vi "Create String for Cluster in Result.vi"(0 "vi reference":refnum<vi>, 2 "output clusters in":string[](array[string]), 5 "ctl refnum":refnum<vi>, 7 "result cluster":refnum<vi>, 11 "error in":errorcluster) -> (4 "output clusters out":string[](array[string]), 15 "error out":errorcluster)   [LabVIEW 2021, in "Converter.lvlib"]
uses:
  Converter.lvlib
  <vilib>/Utility/miscctls.llb/LVPositionTypeDef.ctl
  Converter Reusables/Converter Reusables.lvlib
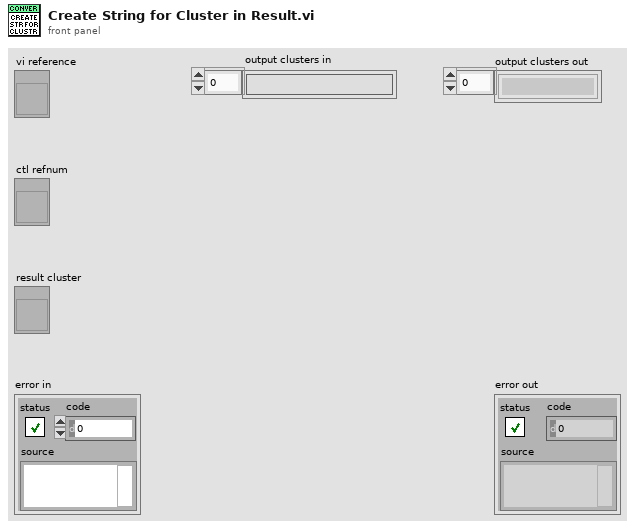
[diagram p1: front panel]
types:
  T1 = typedef "LVPositionTypeDef.ctl" = cluster{"Left":i32, "Top":i32}
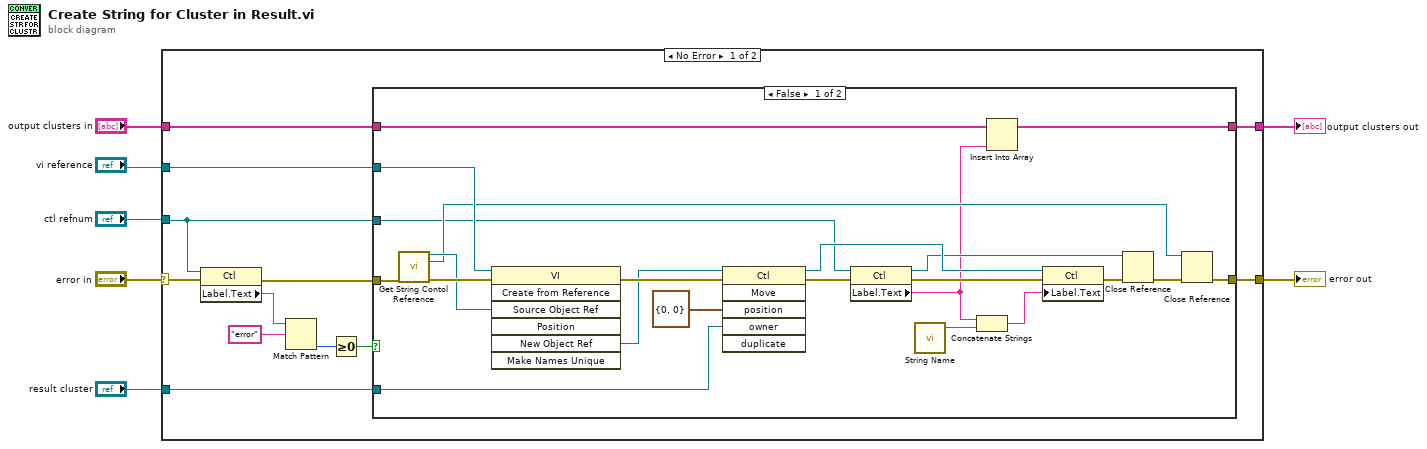
[diagram p0: block diagram]
diagram:
  n1 = case shown="No Error" "error in" {
    selector: "error in" -> [w16 w45]
    tunnel: [w18 w45] -> w1
    tunnel: "vi reference" -> [w19 _]
    tunnel: "result cluster" -> [w8 _]
    tunnel: "ctl refnum" -> [w17 _]
    tunnel: "output clusters in" -> [w12 w44]
    tunnel: [w11 w44] -> w2
    frame No Error {
      n2 = property class="Ctl"(reference=w17, error in=w16) -> (error out=w15:errorcluster, "Label.Text"=w13:string)  [unwired: 1 out]
      n3 = Match Pattern(string=w13, regular expression="error") -> (offset past match=w10:i32)  [unwired: 1 in, 3 out]
      n4 = Greater Or Equal To 0?(x=w10) -> (x >= 0?=w9:bool)
      n5 = case shown="False" w9 {
        tunnel: w19 -> [w40 _]
        tunnel: w8 -> [w39 _]
        tunnel: [w27 w42] -> w18
        tunnel: w17 -> [w25 _]
        tunnel: w15 -> [w24 w42]
        tunnel: w12 -> [w22 w43]
        tunnel: [w21 w43] -> w11
        frame False {
          n6 = call "Get String Contol Reference.vi"("error in"=w24) -> ("string"=w36:refnum<vi>, "vi reference"=w26:refnum<vi>, "error out"=w41:errorcluster)  [unwired: 12 in]
          n7 = invoke class="VI" method="Create from Reference"(reference=w40, error in=w41, "Source Object Ref"=w36) -> (error out=w38:errorcluster, "New Object Ref"=w37:refnum<vi>)  [unwired: 4 in, 5 out]
          n8 = invoke class="Ctl" method="Move"(reference=w37, error in=w38, "position"=T1 {"Left"=0, "Top"=0}, "owner"=w39) -> (reference out=w31:refnum<vi>, error out=w35:errorcluster)  [unwired: 2 in, 4 out]
          n9 = property class="Ctl"(reference=w25, error in=w35) -> (reference out=w29:refnum<vi>, error out=w32:errorcluster, "Label.Text"=w23:string)
          n10 = call "String Name.vi"() -> ("string name"=w34:string)  [unwired: 15 in]
          n11 = Concatenate Strings(w23, w34) -> (w33:string)
          n12 = Insert Into Array(array=w22, new element=w23) -> (w21:string[])  [unwired: 1 in]
          n13 = property class="Ctl"(reference=w31, error in=w32, "Label.Text"=w33) -> (error out=w30:errorcluster)  [unwired: 1 out]
          n14 = Close Reference(reference=w29, error in (no error)=w30) -> (error out=w28:errorcluster)
          n15 = Close Reference(reference=w26, error in (no error)=w28) -> (error out=w27:errorcluster)
        }
        frame True {
        }
      }
    }
    frame Error {
    }
  }
  "error out" <- w1
  "output clusters out" <- w2
